vi "Launch API Tester.vi"(8 "error in (no error)":errorcluster) -> (0 "error out":errorcluster)   [LabVIEW 2022 SP3, in "Serial-Com-Module.lvlib"]
uses:
  Serial-Com-Module.lvlib
  Test Serial-Com-Module API.vi
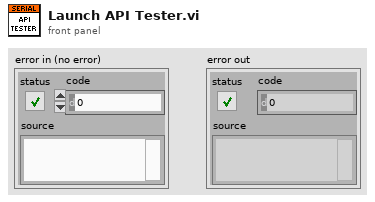
[diagram p1: front panel]
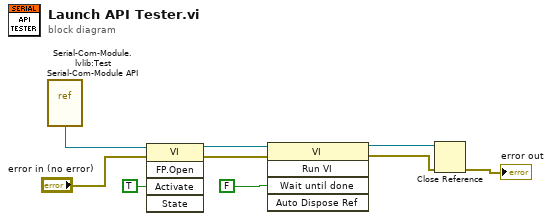
[diagram p0: block diagram]
diagram:
  n1 = vi-ref "Serial-Com-Module.lvlib:Test Serial-Com-Module API.vi"() -> (w4:refnum<vi>)
  n2 = invoke class="VI" method="FP.Open"(reference=w4, error in="error in (no error)", "Activate"=TRUE ("Activate?")) -> (reference out=w6:refnum<vi>, error out=w5:errorcluster)  [unwired: 2 in, 3 out]
  n3 = invoke class="VI" method="Run VI"(reference=w6, error in=w5, "Wait until done"=FALSE ("Wait Until Done")) -> (reference out=w8:refnum<vi>, error out=w7:errorcluster)  [unwired: 2 in, 3 out]
  n4 = Close Reference(reference=w8, error in (no error)=w7) -> (error out=→"error out":errorcluster)
